vi "Do.vi"(8 "error in (no error)":errorcluster, 10 "Actor in":refnum<class "Actor.lvclass">, 11 "Write Controller Enqueuer Msg":refnum<class "Write Controller Enqueuer Msg.lvclass">) -> (0 "error out":errorcluster, 2 "Actor out":refnum<class "Actor.lvclass">)   [LabVIEW 2025, in "Cooler.lvlib" / "Write Controller Enqueuer Msg.lvclass"]
uses:
  Write Controller Enqueuer Msg.lvclass
  <vilib>/ActorFramework/Actor/Actor.lvclass
  Cooler/Cooler.lvclass
  Write Controller Enqueuer Msg.lvclass/Write Controller Enqueuer Msg.ctl
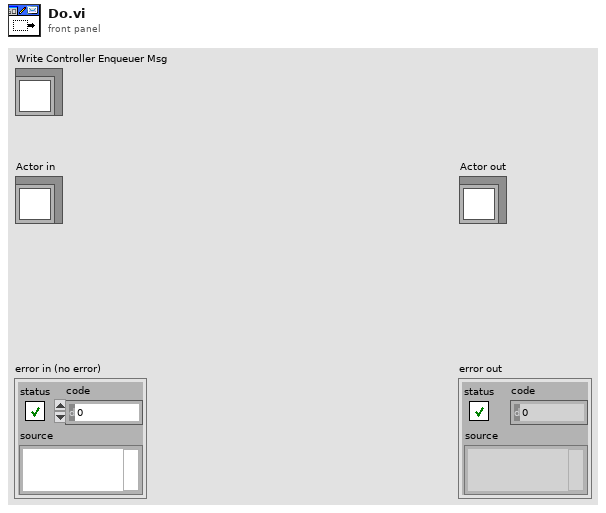
[diagram p1: front panel]
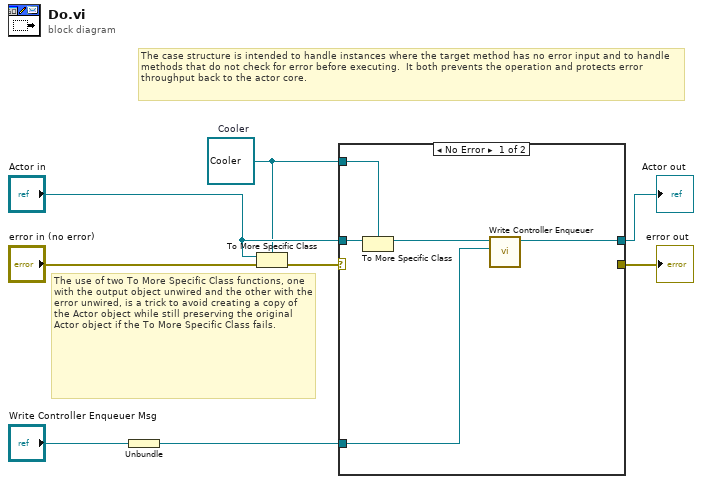
[diagram p0: block diagram]
diagram:
  w2 = refnum<class "Cooler.lvclass"> refnum  # Cooler
  # "The use of two To More Specific Class functions, one with the output object unwired and the other with the error unwired, is a trick to avoid creating a copy of the Actor object while still preserving the original Actor object if the To More Specific Class fails."
  # "The case structure is intended to handle instances where the target method has no error input and to handle methods that do not check for error before executing.  It both prevents the operation and protects error throughput back to the actor core."
  n1 = Unbundle("Write Controller Enqueuer Msg") -> (w1:refnum<class "Message Enqueuer.lvclass">)
  n2 = To More Specific Class(target class=w2, reference="Actor in", error in="error in (no error)") -> (error out=w6:errorcluster)  [unwired: 1 out]
  n3 = case shown="No Error" w6 {
    selector: w6 -> [_ w15]
    tunnel: [_ w15] -> w5
    tunnel: [w13 w14] -> w4
    tunnel: "Actor in" -> [w12 w14]
    tunnel: w2 -> [w11 _]
    tunnel: w1 -> [w9 _]
    frame No Error {
      n4 = To More Specific Class(target class=w11, reference=w12) -> (specific class reference=w10:refnum<class "Cooler.lvclass">)  [unwired: 1 in, 1 out]
      n5 = call "Write Controller Enqueuer.vi"("Controller Enqueuer"=w9, "Cooler in"=w10) -> ("Cooler out"=w13:refnum<class "Cooler.lvclass">)  [unwired: 9 in]
    }
    frame Error {
      # "If type check fails, pass the original object out again."
    }
  }
  "error out" <- w5
  "Actor out" <- w4
